vi "f_Median_SG_filter.vi"(10 "dt":dbl, 11 "Y":dbl[](array[numeric])) -> (3 "output waveform":waveform(dbl))   [LabVIEW 2020]
uses:
  <vilib>/Analysis/3filter.llb/Savitzky-Golay Filter (DBL).vi
  <vilib>/measure/madcrms.llb/Basic Averaged DC-RMS for 1 Chan.vi
  <vilib>/measure/matone.llb/Extract Single Tone Information 1 Chan.vi
  <vilib>/measure/NI_MAPro.lvlib
  <vilib>/Analysis/NI_AALBase.lvlib
panel:
  out "DC value":dbl=1.3484768907563025 format="%0.2p"
  in  "Median rank":i32
  in  "polynomial order":i32=3
  in  "side points":i32=5
  out "detected phase (deg)":dbl=-190.74525534077068 format="%.2p"
  out "detected amplitude":dbl=0.00784016432233465 format="%.2p"
  out "detected frequency":dbl=1.5491635003621782 format="%.2p"
  # "OG = 90"
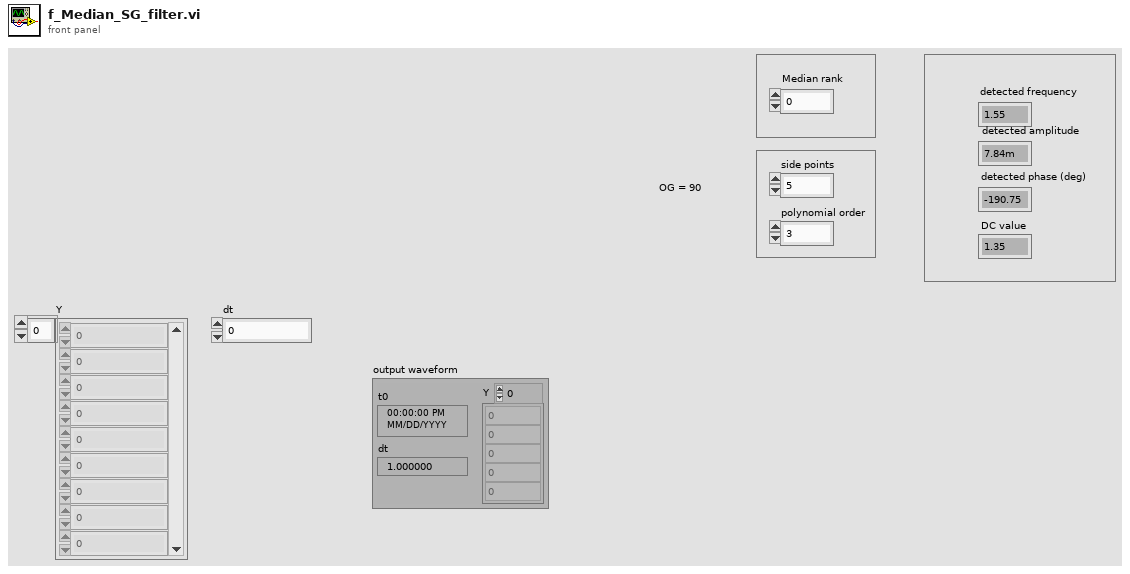
[diagram p1: front panel]
types:
  T1 = enum16{"Rectangular (none)", "Hanning", "Low side lobe"}
  T2 = enum32{"none", "input signal", "detected signal", "residual signal"}
  T3 = cluster{"exported time signal":waveform(dbl), "exported spectrum (dB)":cluster{"f0":dbl, "df":dbl, "dB Spectrum (Hann)":dbl[]}}
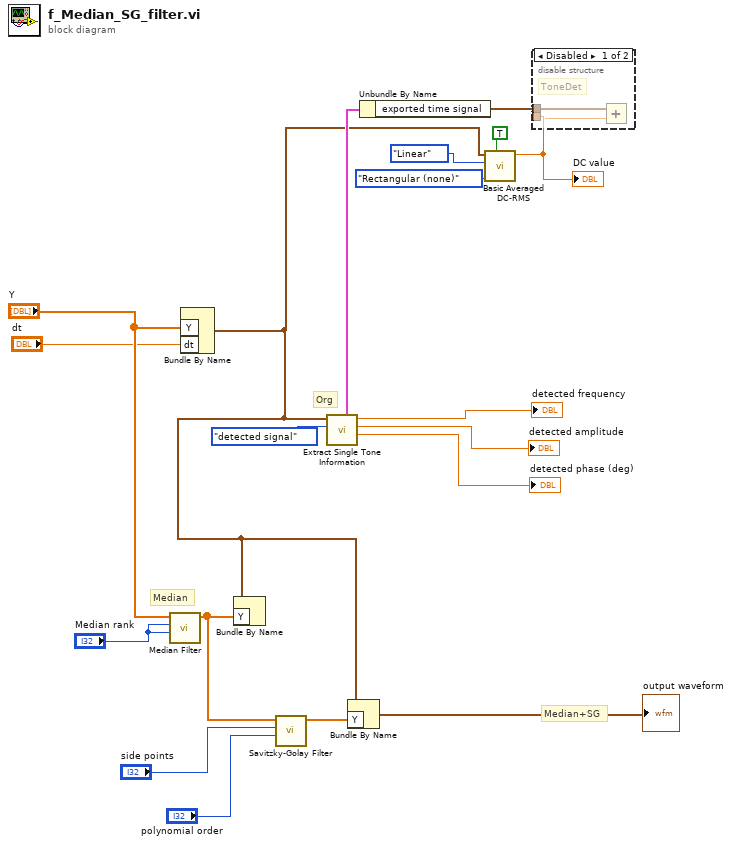
[diagram p0: block diagram]
diagram:
  # "Median"
  # "Median+SG"
  # "Org"
  n1 = call <vilib>:"Median Filter.vi"("right rank"="Median rank", "left rank"="Median rank", "X"="Y") -> ("Filtered X"=w9:dbl[])  [unwired: 7 in, 1 out]
  n2 = Bundle By Name("Y"="Y", "dt"="dt") -> (w3:waveform(dbl))  [unwired: 1 in]
  n3 = Bundle By Name(cluster=w3, "Y"=w9) -> ()  [unwired: 1 out]
  n4 = call-poly <vilib>:"Savitzky-Golay Filter.vi"("polynomial order"="polynomial order", "side points"="side points", "X"=w9) -> ("Filtered X"=w12:dbl[])  [unwired: 7 in, 1 out]
  n5 = call-poly <vilib>:"Extract Single Tone Information.vi"("export mode"=T2."detected signal", "time signal in"=w3) -> ("detected phase (deg)"=→"detected phase (deg)":dbl, "detected amplitude"=→"detected amplitude":dbl, "detected frequency"=→"detected frequency":dbl, "exported signals"=w16:T3)  [unwired: 4 in, 2 out]
  n6 = Bundle By Name(cluster=w3, "Y"=w12) -> (→"output waveform":waveform(dbl))
  n7 = Unbundle By Name(w16) -> ("exported time signal"=w10:waveform(dbl))
  n8 = call-poly <vilib>:"Basic Averaged DC-RMS.vi"("reset"=TRUE, "window"=T1."Rectangular (none)", "averaging type"=enum16{"Linear", "Exponential"}."Linear", "signal in"=w3) -> ("DC value"=w5:dbl)  [unwired: 4 in, 3 out]
  "DC value" <- w5
  n9 = disable-structure shown="Disabled" {
    disable-tunnel: w10 -> [w21 _]
    disable-tunnel: w5 -> [w20 _]
    frame Disabled {
      # "ToneDet"
      n10 = Add(x=w21, y=w20) -> ()  [unwired: 1 out]
    }
    frame Enabled {
    }
  }
